vi "Wait_ms.vi"(8 "error in":errorcluster, 10 "millisec":u32) -> (0 "error in 2":errorcluster)   [LabVIEW 2021]
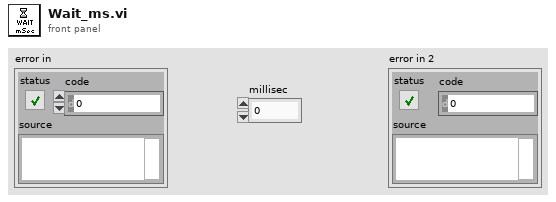
[diagram p1: front panel]
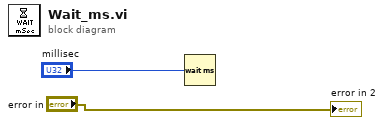
[diagram p0: block diagram]
diagram:
  n1 = Wait (ms)(milliseconds to wait="millisec") -> ()  [unwired: 1 out]
  "error in 2" <- "error in"
